vi "Do UI Exit.vi"(8 "error in (no error)":errorcluster, 11 "Main_UI in":refnum<class "Main_UI.lvclass">) -> (0 "error out":errorcluster, 3 "Main_UI out":refnum<class "Main_UI.lvclass">)   [LabVIEW 2020, in "Main_UI.lvlib" / "Main_UI.lvclass"]
uses:
  Main_UI.lvclass
  <vilib>/event_ctls.llb/usereventprio.ctl
  Main_UI.lvclass/Main_UI.ctl
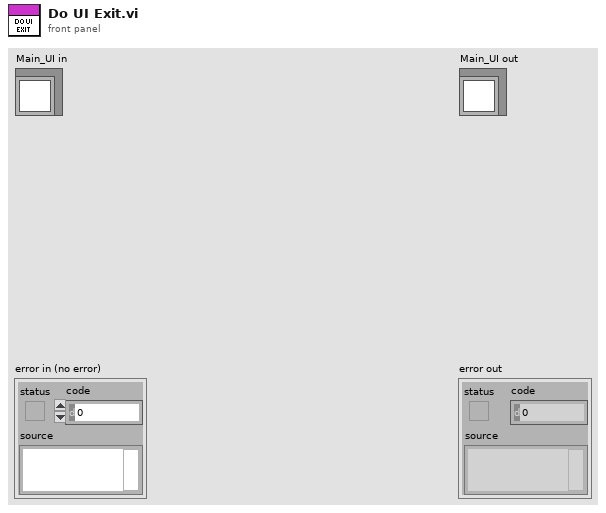
[diagram p1: front panel]
types:
  T1 = typedef "usereventprio.ctl" = enum32{"high priority", "normal priority"}
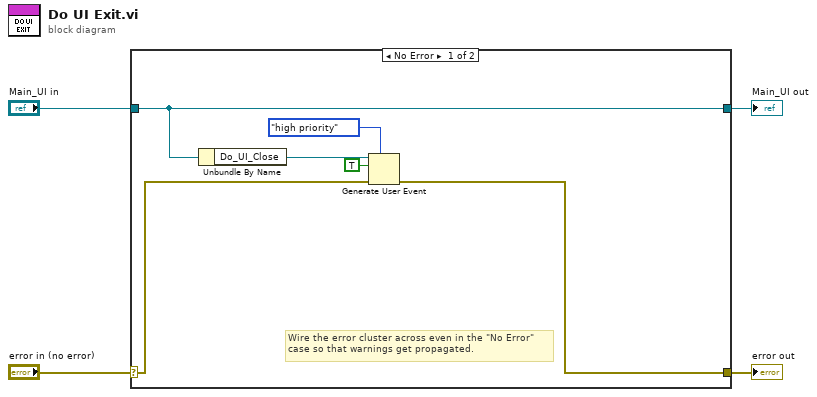
[diagram p0: block diagram]
diagram:
  n1 = case shown="No Error" "error in (no error)" {
    selector: "error in (no error)" -> [w7 w12]
    tunnel: [w6 w12] -> w3
    tunnel: [w10 w11] -> w1
    tunnel: "Main_UI in" -> [w10 w11]
    frame No Error {
      # "Wire the error cluster across even in the \"No Error\"\ncase so that warnings get propagated."
      n2 = Unbundle By Name(w10) -> ("Do_UI_Close"=w9:refnum<user-event>)
      n3 = Generate User Event(priority (normal)=usereventprio."high priority", user event=w9, event data cluster=TRUE ("event data"), error in=w7) -> (error out=w6:errorcluster)  [unwired: 1 out]
    }
    frame Error {
    }
  }
  "error out" <- w3
  "Main_UI out" <- w1
